vi "Write Session.TCPIP.KeepAliveTimeout.vi"(8 "error in (no error)":errorcluster, 10 "Session.TCPIP.KeepAliveTimeout":dbl, 11 "SLSC Interface in":refnum<class "SLSC Interface.lvclass">) -> (0 "error out":errorcluster, 3 "SLSC Interface out":refnum<class "SLSC Interface.lvclass">)   [LabVIEW 2015, in "SLSC Interface.lvclass"]
uses:
  SLSC Interface.lvclass
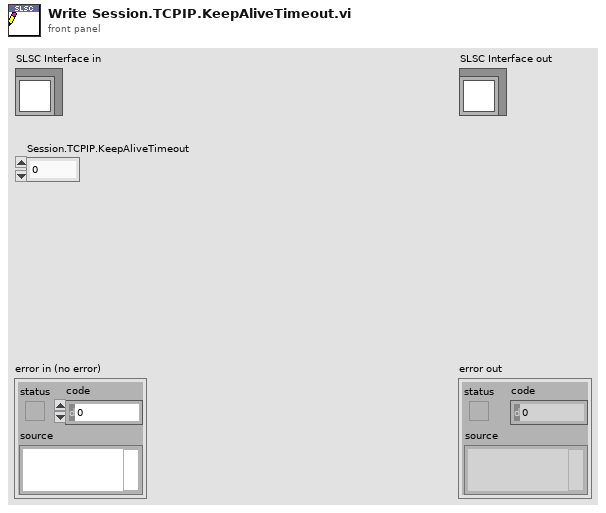
[diagram p1: front panel]
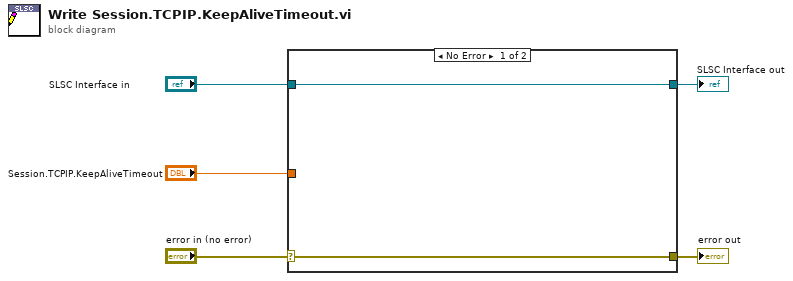
[diagram p0: block diagram]
diagram:
  n1 = case shown="No Error" "error in (no error)" {
    selector: "error in (no error)" -> [w7 w8]
    tunnel: [w7 w8] -> w4
    tunnel: [w6 w9] -> w2
    tunnel: "SLSC Interface in" -> [w6 w9]
    tunnel: "Session.TCPIP.KeepAliveTimeout" -> [_ _]
    frame No Error {
    }
    frame Error {
    }
  }
  "error out" <- w4
  "SLSC Interface out" <- w2
